vi "Close.vi"(8 "error in (no error)":errorcluster, 11 "Measurement Interface in":refnum<class "Measurement Interface.lvclass">) -> (0 "error out":errorcluster, 3 "Measurement Interface out":refnum<class "Measurement Interface.lvclass">)   [LabVIEW 2016, in "Measurement Interface.lvlib" / "Measurement Interface.lvclass"]
uses:
  Measurement Interface.lvclass
  Measurement Interface.lvclass/Measurement Interface.ctl
  Private Methods/Default Steps Database/Read Default Steps Database.vi
  Private Methods/Sequence Call Step/Read Sequence Call Step Dictionary.vi
  Plugins/Sequence Call Step Dictionary.lvlibp/Sequence Call Step Dictionary.lvclass
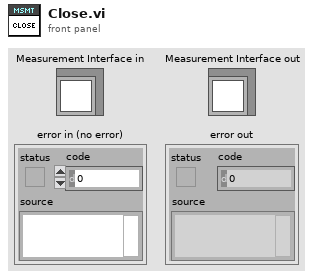
[diagram p1: front panel]
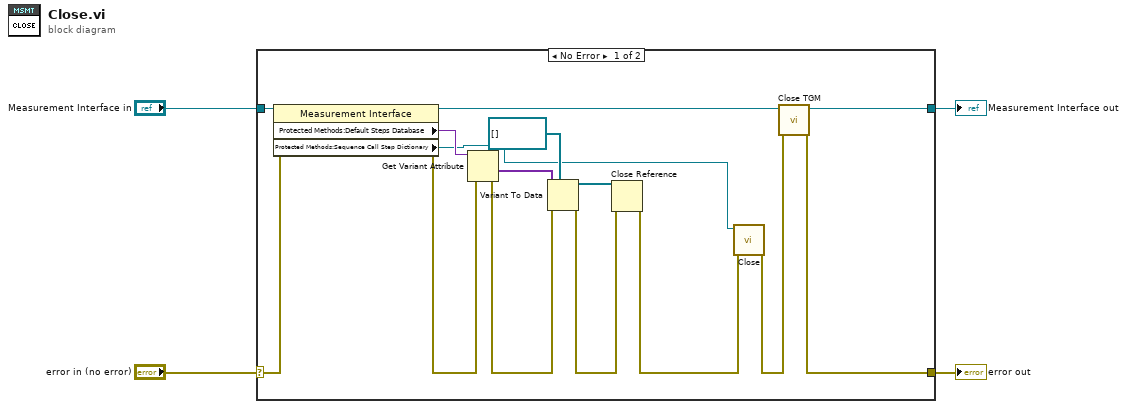
[diagram p0: block diagram]
diagram:
  n1 = case shown="No Error" "error in (no error)" {
    selector: "error in (no error)" -> [w19 w21]
    tunnel: [w7 w21] -> w3
    tunnel: [w5 w20] -> w1
    tunnel: "Measurement Interface in" -> [w18 w20]
    frame No Error {
      n2 = property class="Measurement Interface"(reference=w18, error in=w19) -> (reference out=w6:refnum<class "Measurement Interface.lvclass">, error out=w13:errorcluster, "Protected Methods:Default Steps Database"=w15:variant, "Protected Methods:Sequence Call Step Dictionary"=w10:refnum<class "Sequence Call Step Dictionary.lvclass">)
      n3 = Get Variant Attribute(Variant=w15, error in=w13) -> (values=w17:variant[], error out=w12:errorcluster)  [unwired: 2 in, 2 out]
      n4 = Variant To Data(error in=w12, type=refnum<k7>[] [], Variant=w17) -> (data=w16:refnum<k7>[], error out=w11:errorcluster)
      n5 = Close Reference(reference=w16, error in (no error)=w11) -> (error out=w9:errorcluster)
      n6 = call "Close.vi"("error in (no error)"=w9, "Sequence Call Step Dict in"=w10) -> ("error out"=w8:errorcluster)  [unwired: 9 in]
      n7 = call "Close TGM.vi"("error in (no error)"=w8, "Measurement Interface in"=w6) -> ("error out"=w7:errorcluster, "Measurement Interface out"=w5:refnum<class "Measurement Interface.lvclass">)  [unwired: 8 in]
    }
    frame Error {
    }
  }
  "error out" <- w3
  "Measurement Interface out" <- w1
